vi "MXG_Set_Output_Power.vi"(0 "VISA resource name":refnum<visa-resource-name>, 9 "Output Power\nLevel (dBm)":dbl, 11 "error in":errorcluster) -> (4 "VISA resource name":refnum<visa-resource-name>, 15 "error out":errorcluster)   [LabVIEW 2016]
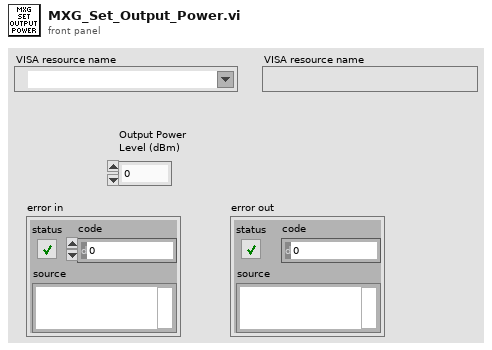
[diagram p1: front panel]
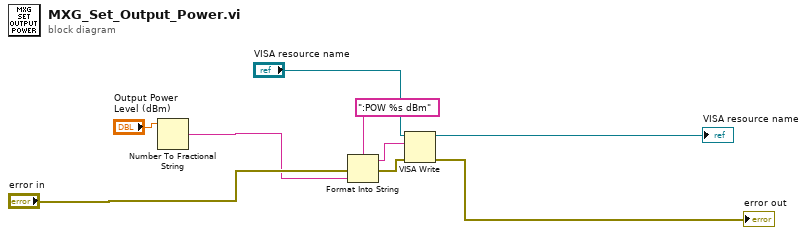
[diagram p0: block diagram]
diagram:
  n1 = Number To Fractional String(number="Output Power\nLevel (dBm)") -> (F-format string=w1:string)  [unwired: 3 in]
  n2 = Format Into String(format string=":POW %s dBm", error in="error in", w1) -> (resulting string=w6:string, error out=w8:errorcluster)  [unwired: 1 in]
  n3 = VISA Write(VISA resource name="VISA resource name", write buffer=w6, error in (no error)=w8) -> (VISA resource name out=→"VISA resource name":refnum<visa-resource-name>, error out=→"error out":errorcluster)  [unwired: 1 out]
